vi "Begin.vi"(8 "error in":errorcluster) -> (0 "error out":errorcluster)   [LabVIEW 2016]
doc: "Called before other user functions, this VI is expected to open initial I/O refnums, load in file data, and do all program initialization. Notice that the <B>error out</B> terminal is simply used for data flow. Wiring it to other structures or subVIs ensures that this VI runs first."
uses:
  <vilib>/Rock Robotics/WPI/DriverStation/WPI_DriverStationRobotMode2.ctl
  Refname/Motors.ctl
  Refname/Controllers.ctl
  <vilib>/Rock Robotics/WPI/Joystick/WPI_JoystickDeviceEnum.ctl
  Refname/Sensors.ctl
  <vilib>/Rock Robotics/WPI/ThirdParty/CanMotor/TalonSRX/WPI_CANTalonSRX_APIControlMode.ctl
  <vilib>/Rock Robotics/WPI/SafetyOutput/WPI_SafetyOutputConfigMenu.ctl
  Refname/Queues.ctl
  <vilib>/Rock Robotics/WPI/ThirdParty/Sensors/Huskie Board/LED Channels.ctl
  <vilib>/Rock Robotics/WPI/ThirdParty/CanMotor/TalonSRX/WPI_CANTalonSRX_APIFeedbackSelect.ctl
  Robot Global Data.vi
  Refname/Refname to String (Sensors).vi
  Refname/Refname to String (Motors).vi
  Refname/Refname to String (Queues).vi
  Refname/Refname to String (Controllers).vi
  <vilib>/Rock Robotics/WPI/ThirdParty/Sensors/ADIS16448 IMU/ADIS16448_IMU.lvlib
  <vilib>/Rock Robotics/SystemInterfaces/spilib/spi_bus.ctl
panel:
  in  "Values to Log":string="TimeStamp, Teleop Called Times, X, Y, Z, a, b, c, d, setpoint 1, setpoint 2, setpoint 3, setpoint 4, wheel power 1, wheel power 2, wheel power 3, wheel power 4"
  in  "PID gains":T1={"proportional gain (Kc)"=5.0, "integral time (Ti, min)"=0.032, "derivative time (Td, min)"=0.0} {"derivative time (Td, min)" format="%.3f"; "integral time (Ti, min)" format="%.8f"; "proportional gain (Kc)" format="%.8f"}
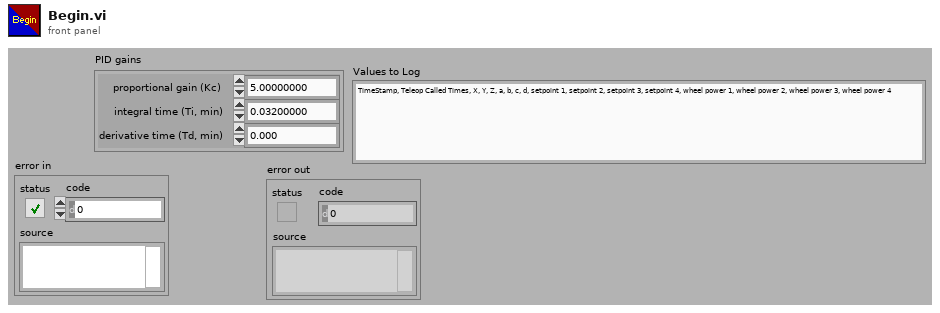
[diagram p1: front panel]
types:
  T1 = cluster{"proportional gain (Kc)":dbl, "integral time (Ti, min)":dbl, "derivative time (Td, min)":dbl}
  T2 = typedef "LED Channels.ctl" = enum8{"SD card D1", "SD card D0", "SD card CLK", "SD card CMD", "SD card D2", "SD card D3", "roboRIO MOSI", "roboRIO MISO", "roboRIO CLK", "roboRIO CS", "roboRIO UART RX", "roboRIO UART TX", "roboRIO SCL", "robotRIO SDA", "HB GPIO 0", "HB GPIO 1", "HB GPIO 2", "HB GPIO 3", "HB LCD", "ADC CS2", "ADC CS1", "ADC DO", "ADC CLK", "ADC DI", "LED 1", "LED 2", "LED 3", "LED 4", "EEPROM SCL", "EEPROM SDA", "USB UART TX", "USB UART RX"}
  T3 = typedef "Queues.ctl" = enum16{"Log Queue"}
  T4 = typedef "WPI_SafetyOutputConfigMenu.ctl" = enum16{"Enable", "Disable"}
  T5 = typedef "Motors.ctl" = enum16{"Wheel 1", "Swerve 1", "Wheel 2", "Swerve 2", "Wheel 3", "Swerve 3", "Wheel 4", "Swerve 4", "Climber"}
  T6 = typedef "WPI_CANTalonSRX_APIControlMode.ctl" = enum8{"Percent VBus", "Speed", "Position", "Slave", "Unchanged / Invalid", "Voltage Compensation", "Current", "Motion Profile", "Motion Magic"}
  T7 = typedef "Sensors.ctl" = enum16{"DIP 1", "DIP 2", "DIP 3", "DIP 4", "IMU", "HuskieBoard"}
  T8 = typedef "WPI_JoystickDeviceEnum.ctl" = enum16{"USB 0", "USB 1", "USB 2", "USB 3", "USB 4", "USB 5"}
  T9 = typedef "Controllers.ctl" = enum16{"Controller 0", "Controller 1"}
  T10 = typedef "WPI_DriverStationRobotMode2.ctl" = enum16{"Autonomous Disabled", "Autonomous Enabled", "Teleop Disabled", "Teleop Enabled", "Disconnected", "Finish", "Test Disabled", "Test Enabled", "Emergency Stopped"}
  T11 = cluster{"connection ID":refnum<k5>, "Running?":bool, "TCP Port":u16, "LastMessageReceivedTime":dbl, "WantsAppRestart":bool, "IsConnect":bool, "Vision Updates":cluster{"CapturedAgoMs":i32, "Valid?":bool, "CapturedAtTimestamp":dbl, "Targets":cluster{"X":dbl, "Y":dbl, "Z":dbl}[]}[]}
  T12 = typedef "WPI_CANTalonSRX_APIFeedbackSelect.ctl" = enum16{"Digital Quadrature Encoder", "Analog Potentiometer", "Analog Encoder", "Count on Quad-A (Rising-Edge)", "Count on Quad-A (Falling-Edge)", "CTR Magnetic Enc (Absolute)", "CTR Magnetic Enc (Relative)", "Pulse Width"}
  T13 = typedef "WPI_MotorControlDeviceRef.ctl" = cluster{"DeviceStatus":errorcluster, "Type":T14, "PWM":cluster{"PWM Channel":T15, "DeadBand":T16}, "CAN":cluster{"Device Number":u8, "SetOutput VI Ref":variant, "GetOutput VI Ref":variant, "Enable VI Ref":variant, "Disable VI Ref":variant, "Data":variant}, "Invert":bool}
  T14 = typedef "WPI_MotorControlType.ctl" = enum16{"PWM", "CAN"}
  T15 = typedef "FPGA_DIOPWMChannel.ctl" = enum8{"PWM 0", "PWM 1", "PWM 2", "PWM 3", "PWM 4", "PWM 5", "PWM 6", "PWM 7", "PWM 8", "PWM 9", "PWM MXP 0", "PWM MXP 1", "PWM MXP 2", "PWM MXP 3", "PWM MXP 4", "PWM MXP 5", "PWM MXP 6", "PWM MXP 7", "PWM MXP 8", "PWM MXP 9", "Invalid"}
  T16 = typedef "WPI_PWMDeadband.ctl" = cluster{"Name":string, "maxPositivePwm":i32, "minPositivePwm":i32, "centerPwm":i32, "maxNegativePwm":i32, "minNegativePwm":i32, "angularRange":u16}
  T17 = typedef "WPI_JoystickDevRef.ctl" = cluster{"Device":T8}
  T18 = typedef "spi_bus.ctl" = enum16{"SPI On-Board, CS0", "SPI On-Board, CS1", "SPI On-Board, CS2", "SPI On-Board, CS3", "SPI MXP", "Invalid"}
  T19 = typedef "ADIS16448_IMU.lvlib/ADI_IMU_ADIS16448_InterruptDevRef.ctl" = cluster{"ADI IMU DevRef":T20, "InterruptRef":T21}
  T20 = typedef "ADIS16448_IMU.lvlib/ADI_IMU_ADIS16448_IMUDevRef.ctl" = cluster{"DevStatus":errorcluster, "Handle":i32, "SPI Bus":T18, "Device Found":bool, "Device Ready":bool, "Yaw Axis":enum16{"X", "Y", "Z"}, "AHRS Algorithm":enum16{"Complementary", "Madgwick"}, "Serial":u16, "Lot ID 2":u16, "Lot ID 1":u16, "Product ID":u16}
  T21 = typedef "WPI_InterruptRef.ctl" = cluster{"DevStatus":errorcluster, "InterruptIndex":T22}
  T22 = typedef "FPGA_InterruptIndex.ctl" = enum8{"0", "1", "2", "3", "4", "5", "6", "7", "Invalid"}
  T23 = typedef "WPI_SerialPortRef.ctl" = cluster{"DevStatus":errorcluster, "Serial Port Name":refnum<visa-resource-name>}
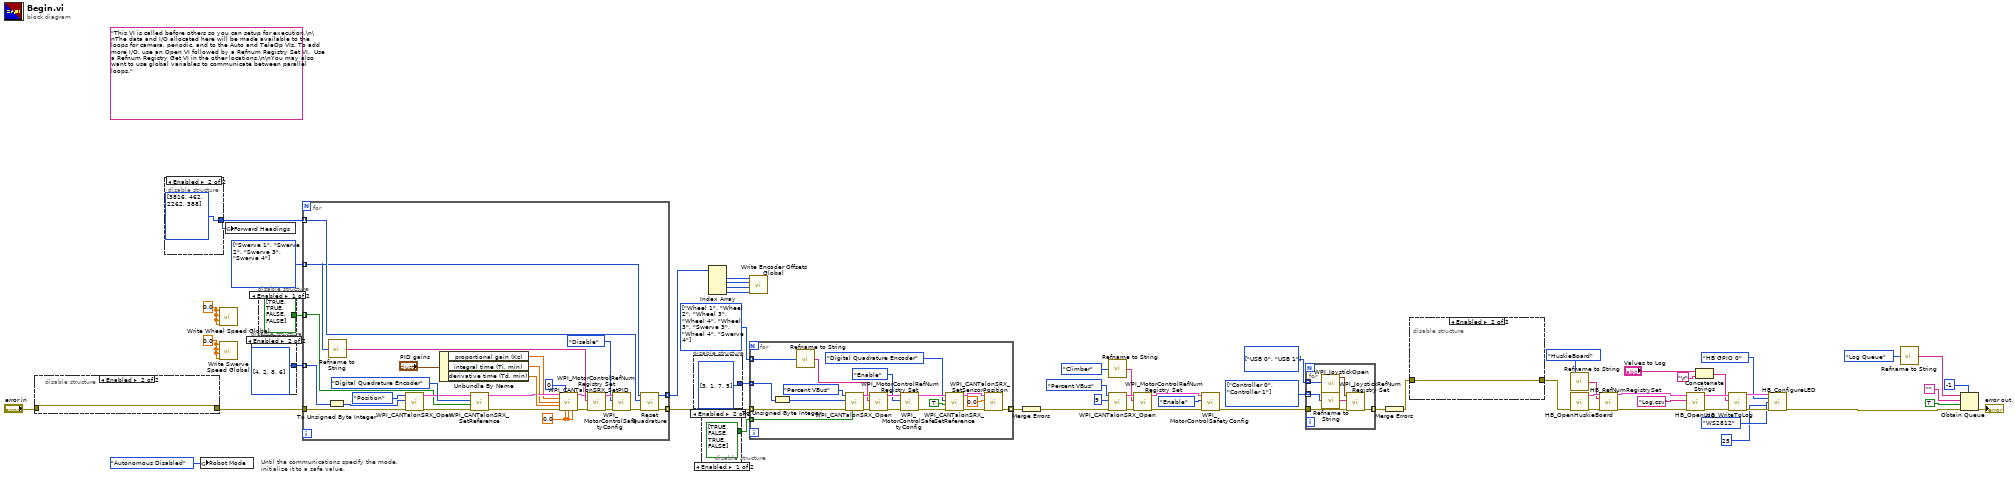
[diagram p0: block diagram]
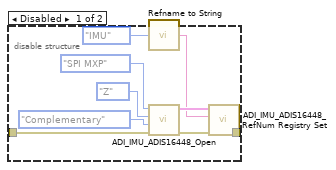
[diagram p2: hidden frame]
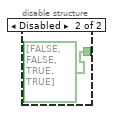
[diagram p3: hidden frame]
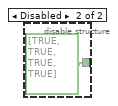
[diagram p4: hidden frame]
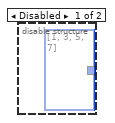
[diagram p5: hidden frame]
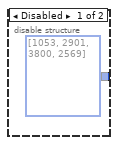
[diagram p6: hidden frame]
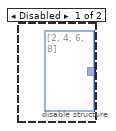
[diagram p7: hidden frame]
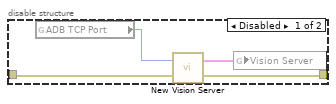
[diagram p8: hidden frame]
diagram:
  w50 = 0.0
  w47 = 0.0
  w54 = T5[] [enum."Swerve 1", enum."Swerve 2", enum."Swerve 3", enum."Swerve 4"] items=["Wheel 1", "Swerve 1", "Wheel 2", "Swerve 2", "Wheel 3", "Swerve 3", "Wheel 4", "Swerve 4", "Climber"]
  w56 = T8[] [enum."USB 0", enum."USB 1"] items=["USB 0", "USB 1", "USB 2", "USB 3", "USB 4", "USB 5"]
  w57 = T9[] [enum."Controller 0", enum."Controller 1"] items=["Controller 0", "Controller 1"]
  w58 = T5[] [enum."Wheel 1", enum."Wheel 2", enum."Wheel 3", enum."Wheel 4", enum."Wheel 3", enum."Swerve 3", enum."Wheel 4", enum."Swerve 4"] items=["Wheel 1", "Swerve 1", "Wheel 2", "Swerve 2", "Wheel 3", "Swerve 3", "Wheel 4", "Swerve 4", "Climber"]
  (unwired) "This VI is called before others so you can setup for execution.\n\nThe data and I/O allocated here will be made available to the loops for camera, periodic, and to the Auto and TeleOp VIs. To add more I/O, use an Open VI followed by a Refnum Registry Set VI.  Use a Refnum Registry Get VI in the other locations.\n\nYou may also want to use global variables to communicate between parallel loops."
  # "Until the communications specify the mode,\ninitialize it to a safe value."
  n1 = disable-structure shown="Enabled" {
    disable-tunnel: [w63 w64] -> w36
    disable-tunnel: "error in" -> [w61 w64]
    frame Disabled {
      n2 = global read "Robot Global Data.vi" "ADB TCP Port"() -> (w60:u16)
      n3 = call "New Vision Server.vi"("error in"=w61, "TCP Port"=w60) -> ("error out"=w63:errorcluster, "Vision Server"=w62:T11)
      n4 = global write "Robot Global Data.vi" "Vision Server"(w62) -> ()
    }
    frame Enabled {
    }
  }
  n5 = disable-structure shown="Enabled" {
    disable-tunnel: [i32[] [1053, 2901, 3800, 2569] i32[] [3816, 462, 2262, 388]] -> w46
    frame Disabled {
    }
    frame Enabled {
    }
  }
  n6 = global write "Robot Global Data.vi" "Robot Mode"(WPI_DriverStationRobotMode2."Autonomous Disabled" ("Robot Mode")) -> ()
  n7 = call "Write Wheel Speed Global.vi"("Wheel 4"=w47, "Wheel 3"=w47, "Wheel 2"=w47, "Wheel 1"=w47) -> ()
  n8 = call "Write Swerve Speed Global.vi"("Swerve 4"=w50, "Swerve 3"=w50, "Swerve 2"=w50, "Swerve 1"=w50) -> ()
  n9 = global write "Robot Global Data.vi" "Forward Headings"(w46) -> ()
  n10 = disable-structure shown="Enabled" {
    disable-tunnel: [i32[] [2, 4, 6, 8] i32[] [4, 2, 8, 6]] -> w53
    frame Disabled {
    }
    frame Enabled {
    }
  }
  n11 = disable-structure shown="Enabled" {
    disable-tunnel: [bool[] [TRUE, TRUE, FALSE, FALSE] bool[] [TRUE, TRUE, TRUE, TRUE]] -> w49
    frame Enabled {
    }
    frame Disabled {
    }
  }
  n12 = for {
    tunnel: w54 -> [w89] mode=indexing
    tunnel: w53 -> [w92] mode=indexing
    tunnel: w36 -> [w91]
    tunnel: w46 -> [w90] mode=indexing
    tunnel: [w87] -> w48 mode=indexing
    tunnel: [w86] -> w51 mode=indexing
    tunnel: w49 -> [w81] mode=indexing
    w78 = 0.0 ("Output")
    n13 = To Unsigned Byte Integer(number=w92) -> (unsigned 8bit integer=w93:u8)
    n14 = call-poly "Refname to String.vi"("Enum"=w89) -> ("String"=w82:string)
    n15 = call <vilib>:"WPI_CANTalonSRX_Open.vi"("error in"=w91, "Device Number"=w93, "Control Mode"=WPI_CANTalonSRX_APIControlMode."Position") -> ("error out"=w83:errorcluster, "CAN Talon SRX Ref"=w84:T13)  [unwired: 7 in]
    n16 = Unbundle By Name("PID gains") -> ("proportional gain (Kc)"=w73:dbl, "integral time (Ti, min)"=w74:dbl, "derivative time (Td, min)"=w79:dbl)
    n17 = call <vilib>:"WPI_CANTalonSRX_SetReference.vi"("error in (no error)"=w83, "Reverse Feedback Sensor"=w81, "Feedback Reference"=WPI_CANTalonSRX_APIFeedbackSelect."Digital Quadrature Encoder", "CAN Talon SRX Ref"=w84) -> ("error out"=w76:errorcluster, "CAN Talon SRX Ref"=w77:T13)  [unwired: 6 in]
    n18 = call <vilib>:"WPI_CANTalonSRX_SetPID.vi"("CAN Talon SRX Ref"=w77, "Parameter Slot"=u8 0, "P"=w73, "I"=w74, "D"=w79, "error in (no error)"=w76, "F"=w78, "I Zone"=w78, "Ramp Rate"=w78) -> ("CAN Talon SRX Ref"=w71:T13, "error out"=w75:errorcluster)  [unwired: 5 in]
    n19 = call <vilib>:"WPI_MotorControlRefNum Registry Set.vi"("error in (no error)"=w75, "refnum name"=w82, "MotorControlDevRef"=w71) -> ("error out"=w96:errorcluster, "MotorControlDevRef"=w95:T13)  [unwired: 7 in]
    n20 = call <vilib>:"WPI_MotorControlSafetyConfig.vi"("error in (no error)"=w96, "mode"=WPI_SafetyOutputConfigMenu."Disable", "MotorControlDevRef"=w95) -> ("error out"=w88:errorcluster)  [unwired: 7 in, 1 out]
    n21 = call "Reset Quadrature.vi"("error in"=w88, "Forward Position"=w90, "Enum"=w89) -> ("error out"=w87:errorcluster, "Encoder Offset"=w86:i32)  [unwired: 7 in]
  }
  n22 = disable-structure shown="Enabled" {
    disable-tunnel: [i32[] [1, 3, 5, 7] i32[] [3, 1, 7, 5]] -> w55
    frame Disabled {
    }
    frame Enabled {
    }
  }
  n23 = disable-structure shown="Enabled" {
    disable-tunnel: [bool[] [TRUE, FALSE, TRUE, FALSE] bool[] [FALSE, FALSE, TRUE, TRUE]] -> w52
    frame Enabled {
    }
    frame Disabled {
    }
  }
  n24 = Index Array(array=w51) -> (element #1=w45:i32, element #2=w44:i32, element #3=w43:i32, element #4=w42:i32)  [unwired: 4 in]
  n25 = call "Write Encoder Offsets Global.vi"("Swerve 4"=w42, "Swerve 3"=w43, "Swerve 2"=w44, "Swerve 1"=w45) -> ()
  n26 = for {
    tunnel: w58 -> [w119] mode=indexing
    tunnel: w55 -> [w111] mode=indexing
    tunnel: [w110] -> w25 mode=indexing
    tunnel: w52 -> [w109] mode=indexing
    tunnel: w48 -> [w108] mode=indexing
    n27 = To Unsigned Byte Integer(number=w111) -> (unsigned 8bit integer=w113:u8)
    n28 = call-poly "Refname to String.vi"("Enum"=w119) -> ("String"=w118:string)
    n29 = call <vilib>:"WPI_CANTalonSRX_Open.vi"("Invert"=w109, "error in"=w108, "Device Number"=w113, "Control Mode"=WPI_CANTalonSRX_APIControlMode."Percent VBus") -> ("error out"=w114:errorcluster, "CAN Talon SRX Ref"=w120:T13)  [unwired: 6 in]
    n30 = call <vilib>:"WPI_MotorControlRefNum Registry Set.vi"("error in (no error)"=w114, "refnum name"=w118, "MotorControlDevRef"=w120) -> ("error out"=w117:errorcluster, "MotorControlDevRef"=w116:T13)  [unwired: 7 in]
    n31 = call <vilib>:"WPI_MotorControlSafetyConfig.vi"("error in (no error)"=w117, "mode"=WPI_SafetyOutputConfigMenu."Enable", "MotorControlDevRef"=w116) -> ("error out"=w105:errorcluster, "MotorControlDevRef"=w104:T13)  [unwired: 7 in]
    n32 = call <vilib>:"WPI_CANTalonSRX_SetReference.vi"("error in (no error)"=w105, "Reverse Feedback Sensor"=TRUE, "Feedback Reference"=WPI_CANTalonSRX_APIFeedbackSelect."Digital Quadrature Encoder", "CAN Talon SRX Ref"=w104) -> ("error out"=w107:errorcluster, "CAN Talon SRX Ref"=w106:T13)  [unwired: 6 in]
    n33 = call <vilib>:"WPI_CANTalonSRX_SetSensorPosition.vi"("error in (no error)"=w107, "New Sensor Position"=0.0, "CAN Talon SRX Ref"=w106) -> ("error out"=w110:errorcluster)  [unwired: 7 in, 1 out]
  }
  n34 = Merge Errors(w25) -> (w26:errorcluster)
  n35 = call-poly "Refname to String.vi"("Enum"=Motors."Climber") -> ("String"=w22:string)
  n36 = call <vilib>:"WPI_CANTalonSRX_Open.vi"("error in"=w26, "Device Number"=u8 9, "Control Mode"=WPI_CANTalonSRX_APIControlMode."Percent VBus") -> ("error out"=w28:errorcluster, "CAN Talon SRX Ref"=w27:T13)  [unwired: 7 in]
  n37 = call <vilib>:"WPI_MotorControlRefNum Registry Set.vi"("error in (no error)"=w28, "refnum name"=w22, "MotorControlDevRef"=w27) -> ("error out"=w30:errorcluster, "MotorControlDevRef"=w29:T13)  [unwired: 7 in]
  n38 = call <vilib>:"WPI_MotorControlSafetyConfig.vi"("error in (no error)"=w30, "mode"=WPI_SafetyOutputConfigMenu."Enable", "MotorControlDevRef"=w29) -> ("error out"=w31:errorcluster)  [unwired: 7 in, 1 out]
  n39 = for {
    tunnel: w57 -> [w127] mode=indexing
    tunnel: w56 -> [w125] mode=indexing
    tunnel: [w123] -> w32 mode=indexing
    tunnel: w31 -> [w122]
    n40 = call <vilib>:"WPI_JoystickOpen.vi"("JoystickDevice"=w125) -> ("JoystickDevRef"=w124:T17)  [unwired: 10 in]
    n41 = call-poly "Refname to String.vi"("Enum"=w127) -> ("string"=w126:string)
    n42 = call <vilib>:"WPI_JoystickRefNum Registry Set.vi"("error in (no error)"=w122, "refnum name"=w126, "JoystickDevRef"=w124) -> ("error out"=w123:errorcluster)  [unwired: 7 in, 1 out]
  }
  n43 = Merge Errors(w32) -> (w33:errorcluster)
  n44 = disable-structure shown="Enabled" {
    disable-tunnel: [w136 w137] -> w34
    disable-tunnel: w33 -> [w133 w137]
    frame Disabled {
      n45 = call-poly "Refname to String.vi"("Enum"=Sensors."IMU") -> ("String"=w129:string)
      n46 = call <vilib>:"ADI_IMU_ADIS16448_Open.vi"("error in"=w133, "AHRS Algorithm"=enum16{"Complementary", "Madgwick"}."Complementary", "Yaw Axis"=enum16{"X", "Y", "Z"}."Z", "SPI Chip Select"=spi_bus."SPI MXP") -> ("error out"=w135:errorcluster, "ADI IMU Interrupt DevRef"=w134:T19)  [unwired: 6 in]
      n47 = call <vilib>:"ADI_IMU_ADIS16448_RefNum Registry Set.vi"("error in (no error)"=w135, "refnum name"=w129, "ADI IMU Interrupt DevRef"=w134) -> ("error out"=w136:errorcluster)  [unwired: 7 in, 1 out]
    }
    frame Enabled {
    }
  }
  n48 = call-poly "Refname to String.vi"("Enum"=Sensors."HuskieBoard") -> ("String"=w38:string)
  n49 = call <vilib>:"HB_OpenHuskieBoard.vi"("error in (no error)"=w34) -> ("error out"=w40:errorcluster, "HBDeviceRef"=w39:T23)  [unwired: 9 in]
  n50 = call <vilib>:"HB_RefNumRegistrySet.vi"("HBDevRef"=w39, "refnum name"=w38, "error in (no error)"=w40) -> ("HBDevRef"=w19:T23, "error out"=w18:errorcluster)  [unwired: 11 in]
  n51 = call <vilib>:"HB_OpenLog.vi"("error in (no error)"=w18, "File Name"="Log.csv", "HBDeviceRef"=w19) -> ("error out"=w12:errorcluster, "HBDeviceRef"=w11:T23)  [unwired: 7 in]
  n52 = Concatenate Strings("Values to Log", "\r") -> (w9:string)
  n53 = call <vilib>:"HB_WriteToLog.vi"("error in (no error)"=w12, "Log string"=w9, "HBDevRef"=w11) -> ("error out"=w5:errorcluster, "HBDevRef"=w6:T23)  [unwired: 7 in]
  n54 = call <vilib>:"HB_ConfigureLED.vi"("HBDevRef"=w6, "LED Strip Channel"=LED_Channels."HB GPIO 0", "LED Model"=enum8{"WS2812", "WS2812B"}."WS2812", "Number of LEDs"=u8 25, "error in (no error)"=w5) -> ("error out"=w1:errorcluster)  [unwired: 9 in, 1 out]
  n55 = call-poly "Refname to String.vi"("Enum"=Queues."Log Queue") -> ("String"=w17:string)
  n56 = Obtain Queue(max queue size (-1, unlimited)=-1, name (unnamed)=w17, element data type="", create if not found? (T)=TRUE, error in (no error)=w1) -> (error out=→"error out":errorcluster)  [unwired: 2 out]
